vi "main-dev.vi"() -> ()   [LabVIEW 2020]
uses:
  controls/digital-output-cluster.ctl
  controls/state-enum.ctl
  controls/digitial-input-cluster.ctl
  controls/analog-input-cluster.ctl
  controls/analog-output-cluster.ctl
  controls/thermocouple-input-cluster.ctl
  controls/adam-5000-serial-settings.ctl
  controls/adam-5000-all-module-datas.ctl
  controls/adam-5000-all-chassis-data.ctl
  controls/adam-5000-chassis-cmd-ack.ctl
  controls/adam-5000-cmd-response.ctl
  controls/adam-5000-chassis-module-types.ctl
  controls/adam-5000-DO-user-input.ctl
  controls/adam-5000-AO-user-input.ctl
  controls/adam-5000-status-indicator-references.ctl
  <vilib>/Instr/_visa.llb/VISA Configure Serial Port (Instr).vi
panel:
  out "cmd-response":T2
  out "Status Indicators":T3
  in  "Debug Mode":bool
  out "1.Thermocouple Inputs (degC)":T4
  in  "5:Digital Outputs":T5
  in  "4:Digital Outputs":T5
  out "0:Analog Inputs":T6
  out "3:Thermocouple Inputs (degC)":T4
  in  "Chassis Settings":T7={"VISA resource name"="COM8", "baud rate (19200)"=19200, "Chassis ID"=1}
  out "Loop Time (mS)":u32
  out "Loop Counter":i32
  out "error IO":errorcluster
  out "error":errorcluster
  in  "exit":bool
  # "ADAM 5000 Controller"
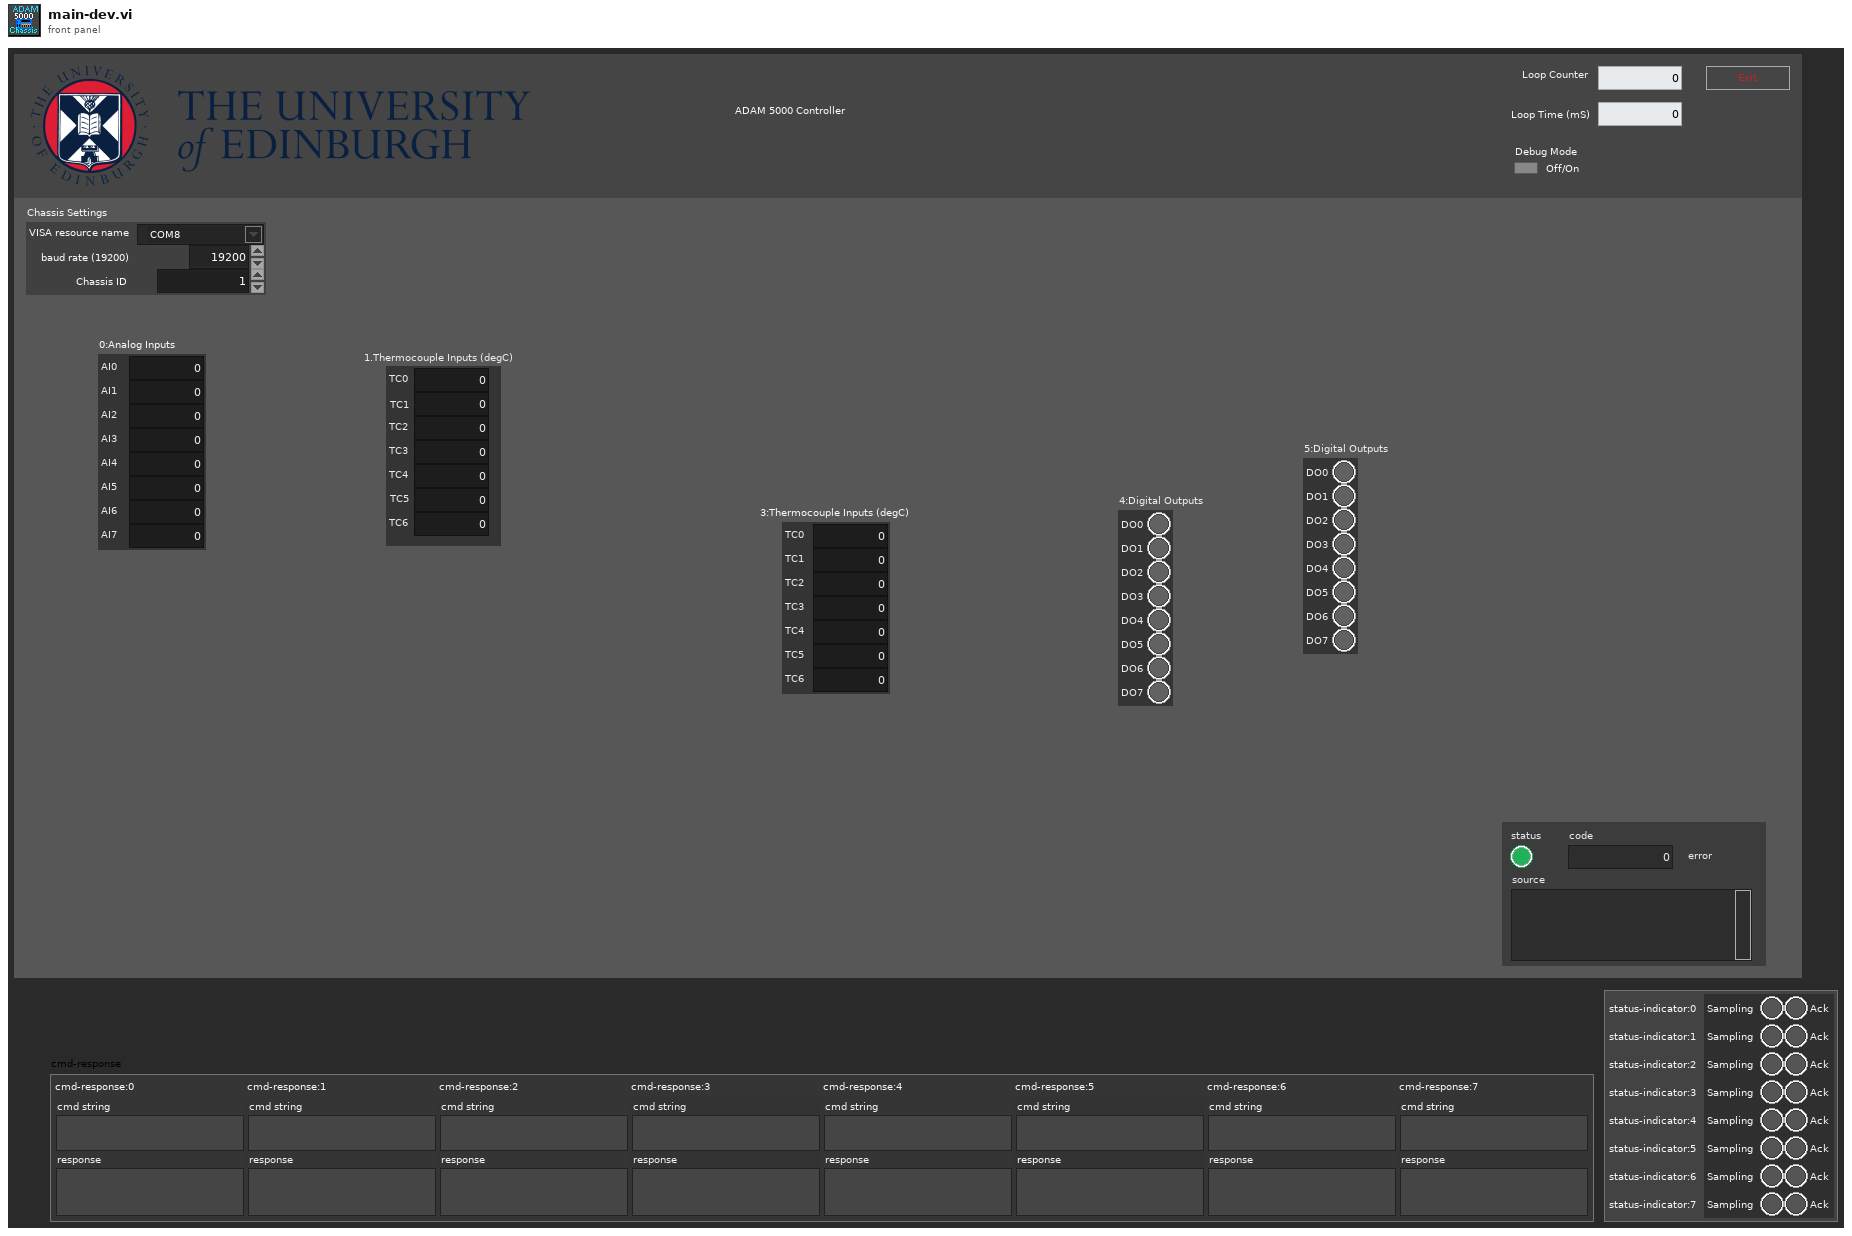
[diagram p1: front panel]
types:
  T1 = typedef "adam-5000-cmd-response.ctl" = cluster{"cmd string":string, "response":string}
  T2 = cluster{"cmd-response:0":T1, "cmd-response:1":T1, "cmd-response:2":T1, "cmd-response:3":T1, "cmd-response:4":T1, "cmd-response:5":T1, "cmd-response:6":T1, "cmd-response:7":T1}
  T3 = cluster{"status-indicator:0":cluster{"Sampling":bool, "Ack":bool}, "status-indicator:1":cluster{"Sampling":bool, "Ack":bool}, "status-indicator:2":cluster{"Sampling":bool, "Ack":bool}, "status-indicator:3":cluster{"Sampling":bool, "Ack":bool}, "status-indicator:4":cluster{"Sampling":bool, "Ack":bool}, "status-indicator:5":cluster{"Sampling":bool, "Ack":bool}, "status-indicator:6":cluster{"Sampling":bool, "Ack":bool}, "status-indicator:7":cluster{"Sampling":bool, "Ack":bool}}
  T4 = typedef "thermocouple-input-cluster.ctl" = cluster{"TC0":dbl, "TC1":dbl, "TC2":dbl, "TC3":dbl, "TC4":dbl, "TC5":dbl, "TC6":dbl}
  T5 = typedef "digital-output-cluster.ctl" = cluster{"DO0":bool, "DO1":bool, "DO2":bool, "DO3":bool, "DO4":bool, "DO5":bool, "DO6":bool, "DO7":bool}
  T6 = typedef "analog-input-cluster.ctl" = cluster{"AI0":dbl, "AI1":dbl, "AI2":dbl, "AI3":dbl, "AI4":dbl, "AI5":dbl, "AI6":dbl, "AI7":dbl}
  T7 = typedef "adam-5000-serial-settings.ctl" = cluster{"VISA resource name":refnum<visa-resource-name>, "baud rate (19200)":u32, "Chassis ID":u8}
  T8 = typedef "adam-5000-chassis-cmd-ack.ctl" = cluster{"cmd-response:0":T1, "cmd-response:1":T1, "cmd-response:2":T1, "cmd-response:3":T1, "cmd-response:4":T1, "cmd-response:5":T1, "cmd-response:6":T1, "cmd-response:7":T1}
  T9 = typedef "adam-5000-all-chassis-data.ctl" = cluster{"slot:0":T10, "slot:1":T10, "slot:2":T10, "slot:3":T10, "slot:4":T10, "slot:5":T10, "slot:6":T10, "slot:7":T10}
  T10 = typedef "adam-5000-all-module-datas.ctl" = cluster{"Digital Outputs":T5, "Digital Inputs":T11, "Analog Outputs":T12, "Analog Inputs":T6, "Thermocouple Inputs (degC)":T4}
  T11 = typedef "digitial-input-cluster.ctl" = cluster{"DI0":bool, "DI1":bool, "DI2":bool, "DI3":bool, "DI4":bool, "DI5":bool, "DI6":bool, "DI7":bool}
  T12 = typedef "analog-output-cluster.ctl" = cluster{"AO0":dbl, "AO1":dbl, "AO2":dbl, "AO3":dbl}
  T13 = typedef "state-enum.ctl" = enum16{"init", "wait", "manual", "start", "run", "reset", "stop", "exit"}
  T14 = enum16{"Digital Output", "Digital Input", "Analog Output", "Analog Input", "Thermocouple", "Power Relay", "empty"}
  T15 = typedef "adam-5000-status-indicator-references.ctl" = cluster{"status-indicator:0":refnum<vi>, "status-indicator:1":refnum<vi>, "status-indicator:2":refnum<vi>, "status-indicator:3":refnum<vi>, "status-indicator:4":refnum<vi>, "status-indicator:5":refnum<vi>, "status-indicator:6":refnum<vi>, "status-indicator:7":refnum<vi>}
  T16 = typedef "adam-5000-AO-user-input.ctl" = cluster{"0:Analog Outputs":T12, "1:Analog Outputs":T12, "2:Analog Outputs":T12, "3:Analog Outputs":T12, "4:Analog Outputs":T12, "5:Analog Outputs":T12, "6:Analog Outputs":T12, "7:Analog Outputs":T12}
  T17 = typedef "adam-5000-DO-user-input.ctl" = cluster{"0:Digital Outputs":T5, "1:Digital Outputs":T5, "2:Digital Outputs":T5, "3:Digital Outputs":T5, "4:Digital Outputs":T5, "5:Digital Outputs":T5, "6:Digital Outputs":T5, "7:Digital Outputs":T5}
  T18 = typedef "adam-5000-chassis-module-types.ctl" = cluster{"Slot 0: Module Type":enum16{"Digital Output", "Digital Input", "Analog Output", "Analog Input", "Thermocouple", "Power Relay", "empty"}, "Slot 1: Module Type":enum16{"Digital Output", "Digital Input", "Analog Output", "Analog Input", "Thermocouple", "Power Relay", "empty"}, "Slot 2: Module Type":enum16{"Digital Output", "Digital Input", "Analog Output", "Analog Input", "Thermocouple", "Power Relay", "empty"}, "Slot 3: Module Type":enum16{"Digital Output", "Digital Input", "Analog Output", "Analog Input", "Thermocouple", "Power Relay", "empty"}, "Slot 4: Module Type":enum16{"Digital Output", "Digital Input", "Analog Output", "Analog Input", "Thermocouple", "Power Relay", "empty"}, "Slot 5: Module Type":enum16{"Digital Output", "Digital Input", "Analog Output", "Analog Input", "Thermocouple", "Power Relay", "empty"}, "Slot 6: Module Type":enum16{"Digital Output", "Digital Input", "Analog Output", "Analog Input", "Thermocouple", "Power Relay", "empty"}, "Slot 7: Module Type":enum16{"Digital Output", "Digital Input", "Analog Output", "Analog Input", "Thermocouple", "Power Relay", "empty"}}
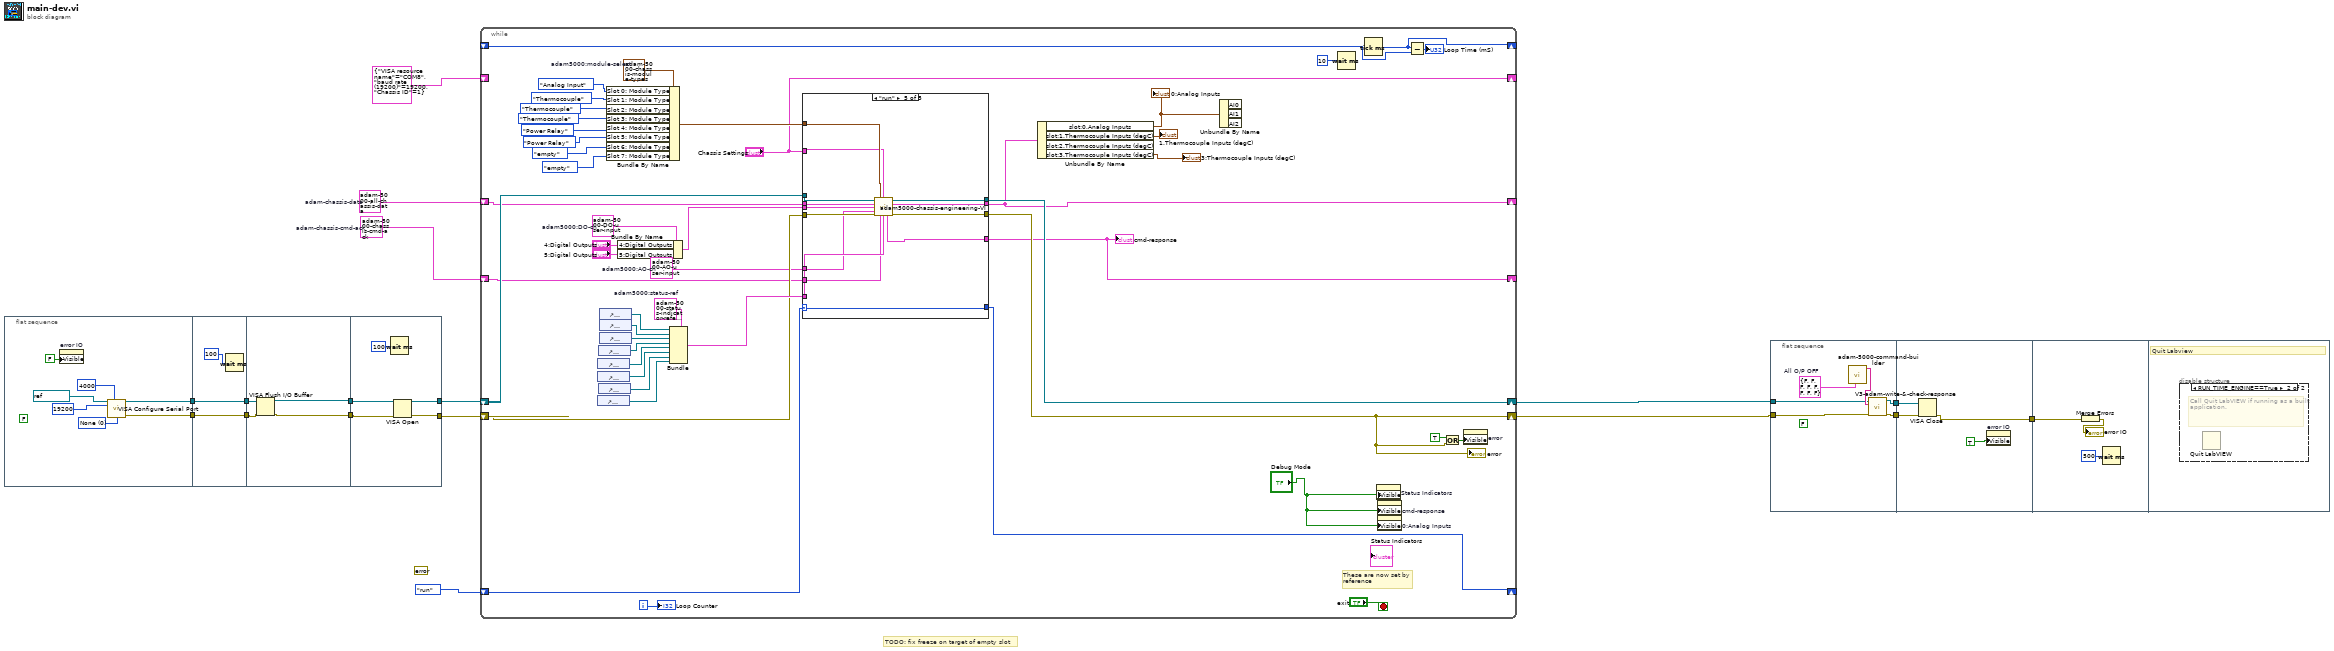
[diagram p0: block diagram]
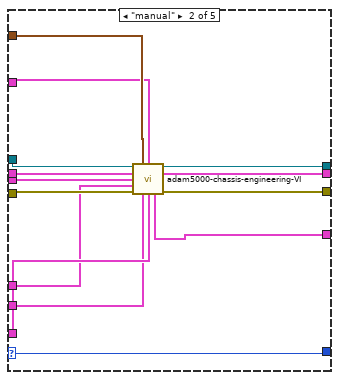
[diagram p4: hidden frame]
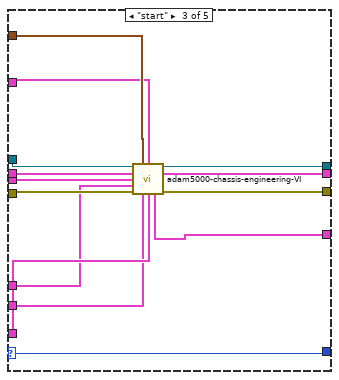
[diagram p5: hidden frame]
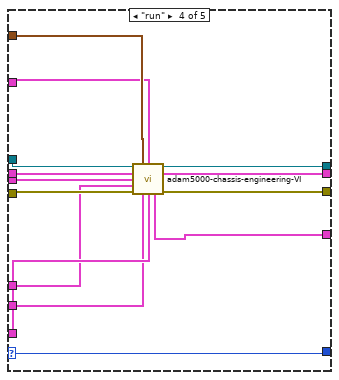
[diagram p6: hidden frame]
diagram:
  w1 = T8 {"cmd-response:0"={"cmd string"="", "response"=""}, "cmd-response:1"={"cmd string"="", "response"=""}, "cmd-response:2"={"cmd string"="", "response"=""}, "cmd-response:3"={"cmd string"="", "response"=""}, "cmd-response:4"={"cmd string"="", "response"=""}, "cmd-response:5"={"cmd string"="", "response"=""}, "cmd-response:6"={"cmd string"="", "response"=""}, "cmd-response:7"={"cmd string"="", "response"=""}}  # adam-chassis-cmd-ack
  w2 = T9 {"slot:0"={"Digital Outputs"={"DO0"=FALSE, "DO1"=FALSE, "DO2"=FALSE, "DO3"=FALSE, "DO4"=FALSE, "DO5"=FALSE, "DO6"=FALSE, "DO7"=FALSE}, "Digital Inputs"={"DI0"=FALSE, "DI1"=FALSE, "DI2"=FALSE, "DI3"=FALSE, "DI4"=FALSE, "DI5"=FALSE, "DI6"=FALSE, "DI7"=FALSE}, "Analog Outputs"={"AO0"=0.0, "AO1"=0.0, "AO2"=0.0, "AO3"=0.0}, "Analog Inputs"={"AI0"=0.0, "AI1"=0.0, "AI2"=0.0, "AI3"=0.0, "AI4"=0.0, "AI5"=0.0, "AI6"=0.0, "AI7"=0.0}, "Thermocouple Inputs (degC)"={"TC0"=0.0, "TC1"=0.0, "TC2"=0.0, "TC3"=0.0, "TC4"=0.0, "TC5"=0.0, "TC6"=0.0}}, "slot:1"={"Digital Outputs"={"DO0"=FALSE, "DO1"=FALSE, "DO2"=FALSE, "DO3"=FALSE, "DO4"=FALSE, "DO5"=FALSE, "DO6"=FALSE, "DO7"=FALSE}, "Digital Inputs"={"DI0"=FALSE, "DI1"=FALSE, "DI2"=FALSE, "DI3"=FALSE, "DI4"=FALSE, "DI5"=FALSE, "DI6"=FALSE, "DI7"=FALSE}, "Analog Outputs"={"AO0"=0.0, "AO1"=0.0, "AO2"=0.0, "AO3"=0.0}, "Analog Inputs"={"AI0"=0.0, "AI1"=0.0, "AI2"=0.0, "AI3"=0.0, "AI4"=0.0, "AI5"=0.0, "AI6"=0.0, "AI7"=0.0}, "Thermocouple Inputs (degC)"={"TC0"=0.0, "TC1"=0.0, "TC2"=0.0, "TC3"=0.0, "TC4"=0.0, "TC5"=0.0, "TC6"=0.0}}, "slot:2"={"Digital Outputs"={"DO0"=FALSE, "DO1"=FALSE, "DO2"=FALSE, "DO3"=FALSE, "DO4"=FALSE, "DO5"=FALSE, "DO6"=FALSE, "DO7"=FALSE}, "Digital Inputs"={"DI0"=FALSE, "DI1"=FALSE, "DI2"=FALSE, "DI3"=FALSE, "DI4"=FALSE, "DI5"=FALSE, "DI6"=FALSE, "DI7"=FALSE}, "Analog Outputs"={"AO0"=0.0, "AO1"=0.0, "AO2"=0.0, "AO3"=0.0}, "Analog Inputs"={"AI0"=0.0, "AI1"=0.0, "AI2"=0.0, "AI3"=0.0, "AI4"=0.0, "AI5"=0.0, "AI6"=0.0, "AI7"=0.0}, "Thermocouple Inputs (degC)"={"TC0"=0.0, "TC1"=0.0, "TC2"=0.0, "TC3"=0.0, "TC4"=0.0, "TC5"=0.0, "TC6"=0.0}}, "slot:3"={"Digital Outputs"={"DO0"=FALSE, "DO1"=FALSE, "DO2"=FALSE, "DO3"=FALSE, "DO4"=FALSE, "DO5"=FALSE, "DO6"=FALSE, "DO7"=FALSE}, "Digital Inputs"={"DI0"=FALSE, "DI1"=FALSE, "DI2"=FALSE, "DI3"=FALSE, "DI4"=FALSE, "DI5"=FALSE, "DI6"=FALSE, "DI7"=FALSE}, "Analog Outputs"={"AO0"=0.0, "AO1"=0.0, "AO2"=0.0, "AO3"=0.0}, "Analog Inputs"={"AI0"=0.0, "AI1"=0.0, "AI2"=0.0, "AI3"=0.0, "AI4"=0.0, "AI5"=0.0, "AI6"=0.0, "AI7"=0.0}, "Thermocouple Inputs (degC)"={"TC0"=0.0, "TC1"=0.0, "TC2"=0.0, "TC3"=0.0, "TC4"=0.0, "TC5"=0.0, "TC6"=0.0}}, "slot:4"={"Digital Outputs"={"DO0"=FALSE, "DO1"=FALSE, "DO2"=FALSE, "DO3"=FALSE, "DO4"=FALSE, "DO5"=FALSE, "DO6"=FALSE, "DO7"=FALSE}, "Digital Inputs"={"DI0"=FALSE, "DI1"=FALSE, "DI2"=FALSE, "DI3"=FALSE, "DI4"=FALSE, "DI5"=FALSE, "DI6"=FALSE, "DI7"=FALSE}, "Analog Outputs"={"AO0"=0.0, "AO1"=0.0, "AO2"=0.0, "AO3"=0.0}, "Analog Inputs"={"AI0"=0.0, "AI1"=0.0, "AI2"=0.0, "AI3"=0.0, "AI4"=0.0, "AI5"=0.0, "AI6"=0.0, "AI7"=0.0}, "Thermocouple Inputs (degC)"={"TC0"=0.0, "TC1"=0.0, "TC2"=0.0, "TC3"=0.0, "TC4"=0.0, "TC5"=0.0, "TC6"=0.0}}, "slot:5"={"Digital Outputs"={"DO0"=FALSE, "DO1"=FALSE, "DO2"=FALSE, "DO3"=FALSE, "DO4"=FALSE, "DO5"=FALSE, "DO6"=FALSE, "DO7"=FALSE}, "Digital Inputs"={"DI0"=FALSE, "DI1"=FALSE, "DI2"=FALSE, "DI3"=FALSE, "DI4"=FALSE, "DI5"=FALSE, "DI6"=FALSE, "DI7"=FALSE}, "Analog Outputs"={"AO0"=0.0, "AO1"=0.0, "AO2"=0.0, "AO3"=0.0}, "Analog Inputs"={"AI0"=0.0, "AI1"=0.0, "AI2"=0.0, "AI3"=0.0, "AI4"=0.0, "AI5"=0.0, "AI6"=0.0, "AI7"=0.0}, "Thermocouple Inputs (degC)"={"TC0"=0.0, "TC1"=0.0, "TC2"=0.0, "TC3"=0.0, "TC4"=0.0, "TC5"=0.0, "TC6"=0.0}}, "slot:6"={"Digital Outputs"={"DO0"=FALSE, "DO1"=FALSE, "DO2"=FALSE, "DO3"=FALSE, "DO4"=FALSE, "DO5"=FALSE, "DO6"=FALSE, "DO7"=FALSE}, "Digital Inputs"={"DI0"=FALSE, "DI1"=FALSE, "DI2"=FALSE, "DI3"=FALSE, "DI4"=FALSE, "DI5"=FALSE, "DI6"=FALSE, "DI7"=FALSE}, "Analog Outputs"={"AO0"=0.0, "AO1"=0.0, "AO2"=0.0, "AO3"=0.0}, "Analog Inputs"={"AI0"=0.0, "AI1"=0.0, "AI2"=0.0, "AI3"=0.0, "AI4"=0.0, "AI5"=0.0, "AI6"=0.0, "AI7"=0.0}, "Thermocouple Inputs (degC)"={"TC0"=0.0, "TC1"=0.0, "TC2"=0.0, "TC3"=0.0, "TC4"=0.0, "TC5"=0.0, "TC6"=0.0}}, "slot:7"={"Digital Outputs"={"DO0"=FALSE, "DO1"=FALSE, "DO2"=FALSE, "DO3"=FALSE, "DO4"=FALSE, "DO5"=FALSE, "DO6"=FALSE, "DO7"=FALSE}, "Digital Inputs"={"DI0"=FALSE, "DI1"=FALSE, "DI2"=FALSE, "DI3"=FALSE, "DI4"=FALSE, "DI5"=FALSE, "DI6"=FALSE, "DI7"=FALSE}, "Analog Outputs"={"AO0"=0.0, "AO1"=0.0, "AO2"=0.0, "AO3"=0.0}, "Analog Inputs"={"AI0"=0.0, "AI1"=0.0, "AI2"=0.0, "AI3"=0.0, "AI4"=0.0, "AI5"=0.0, "AI6"=0.0, "AI7"=0.0}, "Thermocouple Inputs (degC)"={"TC0"=0.0, "TC1"=0.0, "TC2"=0.0, "TC3"=0.0, "TC4"=0.0, "TC5"=0.0, "TC6"=0.0}}}  # adam-chassis-data
  (unwired) errorcluster {"status"=FALSE, "code"=0, "source"=""} ("error")
  # "TODO: fix freeze on target of empty slot"
  n1 = flat-sequence {
    tunnel: [w23] -> w11
    tunnel: [w22] -> w10
    tunnel: w11 -> [w27]
    tunnel: [w27] -> w9
    tunnel: w10 -> [w26]
    tunnel: [w26] -> w8
    tunnel: w9 -> [w31]
    tunnel: [w29] -> w7
    tunnel: w8 -> [w30]
    tunnel: [w28] -> w6
    tunnel: w7 -> [w35]
    tunnel: w6 -> [w34]
    tunnel: [w33] -> w5
    tunnel: [w32] -> w4
    frame #0 {
      w20 = u16 0 items=["None", "XON/XOFF", "RTS/CTS", "XON/XOFF & RTS/CTS", "DTR/DSR", "XON/XOFF & DTR/DSR"] ("flow control (0:none)")
      (unwired) FALSE ("V1")
      n2 = property on="error IO" class="Clust (strict)"("Visible"=FALSE) -> ()  [unwired: 2 in, 2 out]
      n3 = call-poly "VISA Configure Serial Port"("VISA resource name"=refnum<visa-resource-name> "COM8", "timeout (10sec)"=u32 4000, "baud rate (9600)"=u32 19200, "flow control (0:none)"=w20) -> ("VISA resource name out"=w23:refnum<visa-resource-name>, "error out"=w22:errorcluster)  [unwired: 10 in]
    }
    frame #1 {
      n4 = Wait (ms)(milliseconds to wait=u32 100) -> ()  [unwired: 1 out]
    }
    frame #2 {
      n5 = VISA Flush I/O Buffer(VISA resource name=w31, error in (no error)=w30) -> (VISA resource name out=w29:refnum<visa-resource-name>, error out=w28:errorcluster)  [unwired: 1 in]
    }
    frame #3 {
      n6 = Wait (ms)(milliseconds to wait=u32 100) -> ()  [unwired: 1 out]
      n7 = VISA Open(error in (no error)=w34, VISA resource name=w35) -> (VISA resource name=w33:refnum<visa-resource-name>, error out=w32:errorcluster)  [unwired: 3 in]
    }
  }
  n8 = while {
    shift-right: [w37] -> _
    shift-left: state-enum."run" ("state-enum") -> [w38]
    shift-right: [w54] -> w16
    shift-left: w4 -> [w58]
    shift-right: [w79] -> _
    shift-left: _ -> [w81]
    shift-right: ["Chassis Settings"] -> _
    shift-left: T7 {"VISA resource name"="COM8", "baud rate (19200)"=19200, "Chassis ID"=1} ("Chassis Settings") -> [_]
    shift-right: [w57] -> w3
    shift-left: w5 -> [w63]
    shift-right: [w55] -> _
    shift-left: w2 -> [w60]
    shift-right: [w41] -> _
    shift-left: w1 -> [w56]
    i -> [w82]
    stop <- "exit" stop-if-true
    w64 = T15 {"status-indicator:0"=refnum, "status-indicator:1"=refnum, "status-indicator:2"=refnum, "status-indicator:3"=refnum, "status-indicator:4"=refnum, "status-indicator:5"=refnum, "status-indicator:6"=refnum, "status-indicator:7"=refnum}  # adam5000:status-ref
    w42 = T16 {"0:Analog Outputs"={"AO0"=0.0, "AO1"=0.0, "AO2"=0.0, "AO3"=0.0}, "1:Analog Outputs"={"AO0"=0.0, "AO1"=0.0, "AO2"=0.0, "AO3"=0.0}, "2:Analog Outputs"={"AO0"=0.0, "AO1"=0.0, "AO2"=0.0, "AO3"=0.0}, "3:Analog Outputs"={"AO0"=0.0, "AO1"=0.0, "AO2"=0.0, "AO3"=0.0}, "4:Analog Outputs"={"AO0"=0.0, "AO1"=0.0, "AO2"=0.0, "AO3"=0.0}, "5:Analog Outputs"={"AO0"=0.0, "AO1"=0.0, "AO2"=0.0, "AO3"=0.0}, "6:Analog Outputs"={"AO0"=0.0, "AO1"=0.0, "AO2"=0.0, "AO3"=0.0}, "7:Analog Outputs"={"AO0"=0.0, "AO1"=0.0, "AO2"=0.0, "AO3"=0.0}}  # adam5000:AO-ch
    w67 = T17 {"0:Digital Outputs"={"DO0"=FALSE, "DO1"=FALSE, "DO2"=FALSE, "DO3"=FALSE, "DO4"=FALSE, "DO5"=FALSE, "DO6"=FALSE, "DO7"=FALSE}, "1:Digital Outputs"={"DO0"=FALSE, "DO1"=FALSE, "DO2"=FALSE, "DO3"=FALSE, "DO4"=FALSE, "DO5"=FALSE, "DO6"=FALSE, "DO7"=FALSE}, "2:Digital Outputs"={"DO0"=FALSE, "DO1"=FALSE, "DO2"=FALSE, "DO3"=FALSE, "DO4"=FALSE, "DO5"=FALSE, "DO6"=FALSE, "DO7"=FALSE}, "3:Digital Outputs"={"DO0"=FALSE, "DO1"=FALSE, "DO2"=FALSE, "DO3"=FALSE, "DO4"=FALSE, "DO5"=FALSE, "DO6"=FALSE, "DO7"=FALSE}, "4:Digital Outputs"={"DO0"=FALSE, "DO1"=FALSE, "DO2"=FALSE, "DO3"=FALSE, "DO4"=FALSE, "DO5"=FALSE, "DO6"=FALSE, "DO7"=FALSE}, "5:Digital Outputs"={"DO0"=FALSE, "DO1"=FALSE, "DO2"=FALSE, "DO3"=FALSE, "DO4"=FALSE, "DO5"=FALSE, "DO6"=FALSE, "DO7"=FALSE}, "6:Digital Outputs"={"DO0"=FALSE, "DO1"=FALSE, "DO2"=FALSE, "DO3"=FALSE, "DO4"=FALSE, "DO5"=FALSE, "DO6"=FALSE, "DO7"=FALSE}, "7:Digital Outputs"={"DO0"=FALSE, "DO1"=FALSE, "DO2"=FALSE, "DO3"=FALSE, "DO4"=FALSE, "DO5"=FALSE, "DO6"=FALSE, "DO7"=FALSE}}  # adam5000:DO-ch
    w68 = T18 {"Slot 0: Module Type"=enum."Digital Output", "Slot 1: Module Type"=enum."Digital Output", "Slot 2: Module Type"=enum."Digital Output", "Slot 3: Module Type"=enum."Digital Output", "Slot 4: Module Type"=enum."Digital Output", "Slot 5: Module Type"=enum."Digital Output", "Slot 6: Module Type"=enum."Digital Output", "Slot 7: Module Type"=enum."Digital Output"}  # adam5000:module-select
    # "These are now set by\nreference"
    n9 = control-ref of="status-indicator:7"() -> (w69:refnum<vi>)
    n10 = control-ref of="status-indicator:4"() -> (w72:refnum<vi>)
    n11 = control-ref of="status-indicator:5"() -> (w71:refnum<vi>)
    n12 = control-ref of="status-indicator:3"() -> (w73:refnum<vi>)
    n13 = control-ref of="status-indicator:6"() -> (w70:refnum<vi>)
    n14 = control-ref of="status-indicator:2"() -> (w74:refnum<vi>)
    n15 = control-ref of="status-indicator:0"() -> (w76:refnum<vi>)
    n16 = control-ref of="status-indicator:1"() -> (w75:refnum<vi>)
    n17 = Bundle By Name(cluster=w68, "Slot 0: Module Type"=T14."Analog Input", "Slot 1: Module Type"=T14."Thermocouple", "Slot 2: Module Type"=T14."Thermocouple" ("Slot 1: Module Type"), "Slot 3: Module Type"=T14."Thermocouple" ("Slot 1: Module Type"), "Slot 4: Module Type"=T14."Power Relay" ("Slot 1: Module Type"), "Slot 5: Module Type"=T14."Power Relay" ("Slot 1: Module Type"), "Slot 6: Module Type"=T14."empty" ("Slot 1: Module Type"), "Slot 7: Module Type"=T14."empty" ("Slot 1: Module Type")) -> (w62:T18)
    n18 = Bundle By Name(cluster=w67, "4:Digital Outputs"="4:Digital Outputs", "5:Digital Outputs"="5:Digital Outputs") -> (w61:T17)
    n19 = Bundle(cluster=w64, "status-indicator:0"=w76, "status-indicator:1"=w75, "status-indicator:2"=w74, "status-indicator:3"=w73, "status-indicator:4"=w72, "status-indicator:5"=w71, "status-indicator:6"=w70, "status-indicator:7"=w69) -> (w59:T15)
    n20 = case shown="\"run\"" w38 {
      selector: w38 -> [w89 w90 w104 w118 w132]
      tunnel: w63 -> [w87 w103 w117 w131 w145]
      tunnel: w62 -> [_ w102 w116 w130 w144]
      tunnel: w61 -> [_ w101 w115 w129 w143]
      tunnel: w60 -> [w88 w100 w114 w128 w142]
      tunnel: w59 -> [_ w99 w113 w127 w141]
      tunnel: w58 -> [w86 w98 w112 w126 w140]
      tunnel: [w87 w97 w111 w125 w139] -> w57
      tunnel: w56 -> [w85 w96 w110 w124 w138]
      tunnel: [w88 w95 w109 w123 w137] -> w55
      tunnel: [w86 w94 w108 w122 w136] -> w54
      tunnel: "Chassis Settings" -> [_ w93 w107 w121 w135]
      tunnel: w42 -> [_ w92 w106 w120 w134]
      tunnel: [w85 w91 w105 w119 w133] -> w41
      tunnel: [w89 w90 w104 w118 w132] -> w37
      frame "init", Default {
      }
      frame "manual" {
        n21 = call "adam5000-chassis-engineering-VI.vi"("VISA Refnum in"=w103, "adam5000:module-type-select"=w102, "Chassis Settings in"=w93, "adam5000:all-data-in"=w100, "adam5000:DO-ch"=w101, "adam5000:AO-ch"=w92, "error in (no error)"=w98, "adam-chassis-cmd-ack"=w96, "adam5000:status-ref"=w99) -> ("VISA Refnum out"=w97:refnum<visa-resource-name>, "adam5000:all-data-out"=w95:T9, "adam-chassis-cmd-response-out"=w91:T8, "error out"=w94:errorcluster)  [unwired: 3 in]
      }
      frame "start" {
        n22 = call "adam5000-chassis-engineering-VI.vi"("VISA Refnum in"=w117, "adam5000:module-type-select"=w116, "Chassis Settings in"=w107, "adam5000:all-data-in"=w114, "adam5000:DO-ch"=w115, "adam5000:AO-ch"=w106, "error in (no error)"=w112, "adam-chassis-cmd-ack"=w110, "adam5000:status-ref"=w113) -> ("VISA Refnum out"=w111:refnum<visa-resource-name>, "adam5000:all-data-out"=w109:T9, "adam-chassis-cmd-response-out"=w105:T8, "error out"=w108:errorcluster)  [unwired: 3 in]
      }
      frame "run" {
        n23 = call "adam5000-chassis-engineering-VI.vi"("VISA Refnum in"=w131, "adam5000:module-type-select"=w130, "Chassis Settings in"=w121, "adam5000:all-data-in"=w128, "adam5000:DO-ch"=w129, "adam5000:AO-ch"=w120, "error in (no error)"=w126, "adam-chassis-cmd-ack"=w124, "adam5000:status-ref"=w127) -> ("VISA Refnum out"=w125:refnum<visa-resource-name>, "adam5000:all-data-out"=w123:T9, "adam-chassis-cmd-response-out"=w119:T8, "error out"=w122:errorcluster)  [unwired: 3 in]
      }
      frame "run" {
        n24 = call "adam5000-chassis-engineering-VI.vi"("VISA Refnum in"=w145, "adam5000:module-type-select"=w144, "Chassis Settings in"=w135, "adam5000:all-data-in"=w142, "adam5000:DO-ch"=w143, "adam5000:AO-ch"=w134, "error in (no error)"=w140, "adam-chassis-cmd-ack"=w138, "adam5000:status-ref"=w141) -> ("VISA Refnum out"=w139:refnum<visa-resource-name>, "adam5000:all-data-out"=w137:T9, "adam-chassis-cmd-response-out"=w133:T8, "error out"=w136:errorcluster)  [unwired: 3 in]
      }
    }
    "error" <- w54
    "cmd-response" <- w41
    n25 = Unbundle By Name(w55) -> ("slot:0.Analog Inputs"=w39:T6, "slot:1.Thermocouple Inputs (degC)"=→"1.Thermocouple Inputs (degC)":T4, "slot:3.Thermocouple Inputs (degC)"=→"3:Thermocouple Inputs (degC)":T4)  [unwired: 1 out]
    "0:Analog Inputs" <- w39
    n26 = Unbundle By Name(w39) -> ()  [unwired: 3 out]
    n27 = Wait (ms)(milliseconds to wait=u32 10) -> ()  [unwired: 1 out]
    n28 = Tick Count (ms)() -> (millisecond timer value=w79:u32)
    n29 = property on="Status Indicators" class="Clust (strict)"("Visible"="Debug Mode") -> ()  [unwired: 2 in, 2 out]
    n30 = property on="cmd-response" class="Clust (strict)"("Visible"="Debug Mode") -> ()  [unwired: 2 in, 2 out]
    n31 = property on="0:Analog Inputs" class="Clust (strict)"("Visible"="Debug Mode") -> ()  [unwired: 2 in, 2 out]
    n32 = Subtract(x=w79, y=w81) -> (x-y=→"Loop Time (mS)":u32)
    n33 = Or(x=TRUE ("Debug Mode"), y=w54) -> (x .or. y?=w78:bool)
    n34 = property on="error" class="Clust (strict)"("Visible"=w78) -> ()  [unwired: 2 in, 2 out]
    "Loop Counter" <- w82
  }
  n35 = flat-sequence {
    tunnel: w16 -> [w150]
    tunnel: [w149] -> w14
    tunnel: [w148] -> w13
    tunnel: w3 -> [w146]
    tunnel: [w152] -> w15
    tunnel: w14 -> [w153]
    tunnel: w13 -> [w154]
    tunnel: w15 -> [w156]
    frame #0 {
      (unwired) FALSE ("V1")
      w147 = T5 {"DO0"=FALSE, "DO1"=FALSE, "DO2"=FALSE, "DO3"=FALSE, "DO4"=FALSE, "DO5"=FALSE, "DO6"=FALSE, "DO7"=FALSE}  # All O/P OFF
      n36 = call "adam-5000-command-builder.vi"("Output Control"=w147) -> ("Command Out"=w151:string)  [unwired: 8 in, 2 out]
      n37 = call "V3-adam-write-&-check-response.vi"("error in (no error)"=w150, "write buffer"=w151, "VISA resource name"=w146) -> ("error out"=w148:errorcluster, "VISA resource name out"=w149:refnum<visa-resource-name>)  [unwired: 4 in, 3 out]
    }
    frame #1 {
      n38 = VISA Close(VISA resource name=w153, error in (no error)=w154) -> (error out=w152:errorcluster)
      n39 = property on="error IO" class="Clust (strict)"("Visible"=TRUE) -> ()  [unwired: 2 in, 2 out]
    }
    frame #2 {
      n40 = Merge Errors(w156) -> (→"error IO":errorcluster)
      n41 = Wait (ms)(milliseconds to wait=u32 500) -> ()  [unwired: 1 out]
    }
    frame #3 {
      # "Quit Labview"
      n42 = disable-structure "Conditional Disable Structure" shown="RUN_TIME_ENGINE==True" {
        frame condition #0 (active) {
        }
        frame condition #1 {
          # "Call Quit LabVIEW if running as a built application."
          n43 = Quit LabVIEW() -> ()  [unwired: 1 in]
        }
      }
    }
  }
